vi "GVZwangs.vi"() -> ()   [LabVIEW 2010]
panel:
  in  "ZwangsLangsameHeizungenSP!":dbl[](array[numeric])
  out "ZwangsLangsameHeizungenSP?":bool[](array[boolean])
  out "ZwangsSchnelleHeizungen?":bool[](array[boolean])
  in  "ZwangsSchnelleHeizungen!":dbl[](array[numeric])
  out "ZwangsFPGABoolesch!":bool[](array[boolean])
  out "ZwangsFPGABoolesch?":bool[](array[boolean])
  out "ZwangsLangsameHeizungenAn!":bool[](array[boolean])
  out "ZwangsLangsameHeizungenAn?":bool[](array[boolean])
  out "ZwangsDIO!":cluster{bool[]}[](array[cluster])
  out "ZwangsDIO?":cluster{bool[]}[](array[cluster])
  out "ZwangsHorst!":cluster{dbl[]}[](array[cluster])
  out "ZwangsHorst?":cluster{bool[]}[](array[cluster])
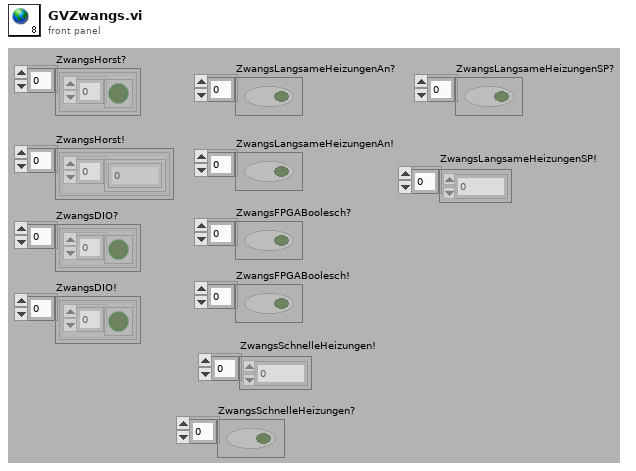
[diagram p1: front panel]
diagram:
